vi "Read IProjectItemFactory.vi"(11 "ProjectItem in":refnum<class "Search.lvclass">) -> (2 "IProjectItemFactory":refnum<class "IProjectItemFactory.lvclass">, 3 "ProjectItem out":refnum<class "Search.lvclass">)   [LabVIEW 2016, in "Search.lvclass"]
uses:
  Search.lvclass
  IProjectItemFactory/IProjectItemFactory.lvclass
  Search.lvclass/Search.ctl
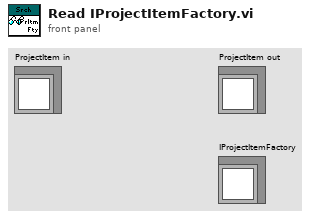
[diagram p1: front panel]
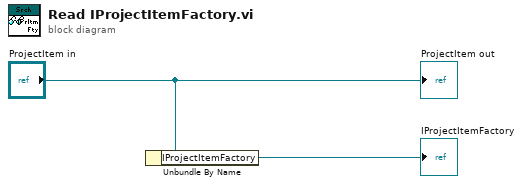
[diagram p0: block diagram]
diagram:
  n1 = Unbundle By Name("ProjectItem in") -> ("IProjectItemFactory"=→"IProjectItemFactory":refnum<class "IProjectItemFactory.lvclass">)
  "ProjectItem out" <- "ProjectItem in"
